vi "ASCII Coding.vi"(1 "cmd":string) -> (0 "cmd sent":string)   [LabVIEW 2012]
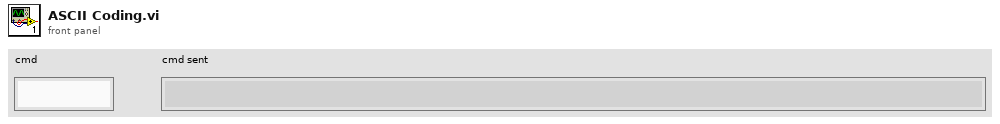
[diagram p1: front panel]
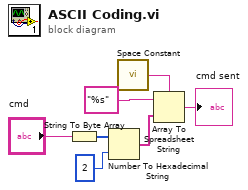
[diagram p0: block diagram]
diagram:
  n1 = String To Byte Array(string="cmd") -> (unsigned byte array=w3:u8[])
  n2 = Number To Hexadecimal String(1:i16 2 ("width (-)"), 2:w3) -> (0:w1:string[])
  n3 = call <vilib>:"Space Constant.vi"() -> ("String"=w6:string)
  n4 = Array To Spreadsheet String(delimiter (Tab)=w6, array=w1, 3:"%s" ("format string")) -> (spreadsheet string=→"cmd sent":string)
